vi "strip newline.vi"(10 "offset":i32, 11 "\\r\\n terminated string":string) -> (3 "striped string":string)   [LabVIEW 2019, in "RESP3.lvlib"]
uses:
  RESP3.lvlib
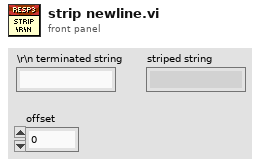
[diagram p1: front panel]
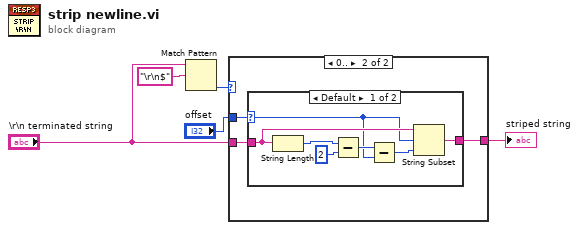
[diagram p0: block diagram]
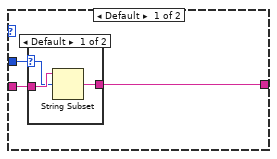
[diagram p2: hidden frame]
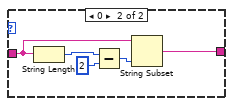
[diagram p4: hidden frame]
diagram:
  n1 = Match Pattern(string="\\r\\n terminated string", regular expression="\r\n$") -> (offset past match=w4:i32)  [unwired: 1 in, 3 out]
  n2 = case shown="0.." w4 {
    tunnel: "offset" -> [w8 w15]
    tunnel: "\\r\\n terminated string" -> [w7 w14]
    tunnel: [w6 w13] -> w1
    frame Default {
      n3 = case shown="Default" w8 {
        selector: w8 -> [w10 _]
        tunnel: w7 -> [w11 w12]
        tunnel: [w9 w12] -> w6
        frame Default {
          n4 = String Subset(string=w11, offset (0)=w10) -> (substring=w9:string)  [unwired: 1 in]
        }
        frame 0 {
        }
      }
    }
    frame 0.. {
      n5 = case shown="Default" w15 {
        selector: w15 -> [w18 _]
        tunnel: w14 -> [w20 w27]
        tunnel: [w16 w23] -> w13
        frame Default {
          n6 = String Length(string=w20) -> (length=w22:i32)
          n7 = Subtract(x=w22, y=2) -> (x-y=w19:i32)
          n8 = Subtract(x=w19, y=w18) -> (x-y=w17:i32)
          n9 = String Subset(string=w20, offset (0)=w18, length (rest)=w17) -> (substring=w16:string)
        }
        frame 0 {
          n10 = String Length(string=w27) -> (length=w26:i32)
          n11 = Subtract(x=w26, y=2) -> (x-y=w24:i32)
          n12 = String Subset(string=w27, length (rest)=w24) -> (substring=w23:string)  [unwired: 1 in]
        }
      }
    }
  }
  "striped string" <- w1
